vi "ChannelSim.vi"(3 "Receiver Queue":refnum<queue>, 4 "Channel Array In":T2(array[cluster]), 5 "index":i32) -> (0 "error out":errorcluster)   [LabVIEW 2014]
panel:
  out "data":T1
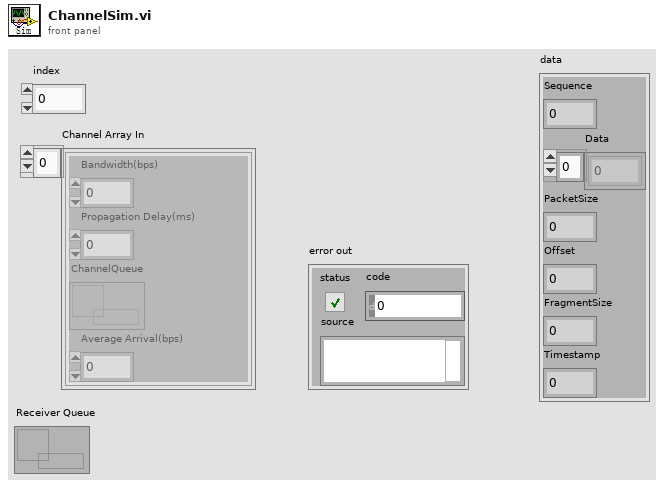
[diagram p1: front panel]
types:
  T1 = cluster{"Sequence":i32, "Data":u8[], "PacketSize":i32, "Offset":i32, "FragmentSize":i32, "Timestamp":i32}
  T2 = cluster{"Bandwidth(bps)":i32, "Propagation Delay(ms)":i32, "ChannelQueue":refnum<queue>, "Average Arrival(bps)":dbl}[]
  T3 = cluster{"Bandwidth(bps)":i32, "Propagation Delay(ms)":i32, "ChannelQueue":refnum<queue>, "Average Arrival(bps)":dbl}
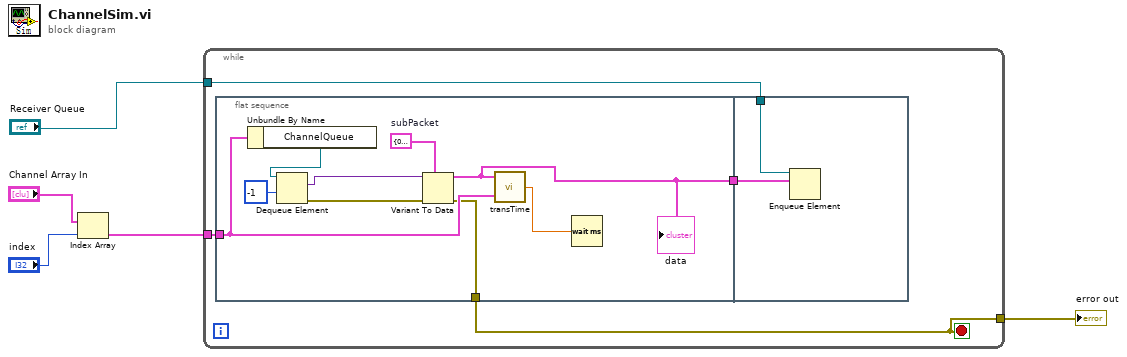
[diagram p0: block diagram]
diagram:
  n1 = Index Array(array="Channel Array In", index="index") -> (element=w4:T3)
  n2 = while {
    tunnel: w4 -> [w9]
    tunnel: "Receiver Queue" -> [w8]
    tunnel: [w7] -> w2
    stop <- w7 stop-if-true
    n3 = flat-sequence {
      tunnel: w9 -> [w15]
      tunnel: [w13] -> w7
      tunnel: [w11] -> w6
      tunnel: w8 -> [w20]
      tunnel: w6 -> [w19]
      frame #0 {
        w12 = T1 {"Sequence"=0, "Data"=[], "PacketSize"=0, "Offset"=0, "FragmentSize"=0, "Timestamp"=0}  # subPacket
        n4 = Unbundle By Name(w15) -> ("ChannelQueue"=w18:refnum<queue>)
        n5 = Dequeue Element(queue=w18, timeout in ms (-1)=-1) -> (element=w16:variant, error out=w17:errorcluster)  [unwired: 1 in, 2 out]
        n6 = Variant To Data(error in=w17, type=w12, Variant=w16) -> (data=w11:T1, error out=w13:errorcluster)
        "data" <- w11
        n7 = call "transTime.vi"("Channel"=w15, "subPacket"=w11) -> ("delay"=w14:dbl)
        n8 = Wait (ms)(milliseconds to wait=w14) -> ()  [unwired: 1 out]
      }
      frame #1 {
        n9 = Enqueue Element(queue=w20, element=w19) -> ()  [unwired: 2 in, 3 out]
      }
    }
  }
  "error out" <- w2
